vi "transmit.vi"(8 "error in (no error)":errorcluster, 11 "DesktopModbus in":refnum<class "DesktopModbus.lvclass">) -> (0 "error out":errorcluster, 3 "DesktopModbus out":refnum<class "DesktopModbus.lvclass">)   [LabVIEW 2015, in "DesktopModbus.lvclass"]
uses:
  DesktopModbus.lvclass
  Common_RT_Modbus/DataTypes/Frame.ctl
  DesktopModbus.lvclass/DesktopModbus.ctl
  Common_RT_Modbus/RTModbus.lvlib
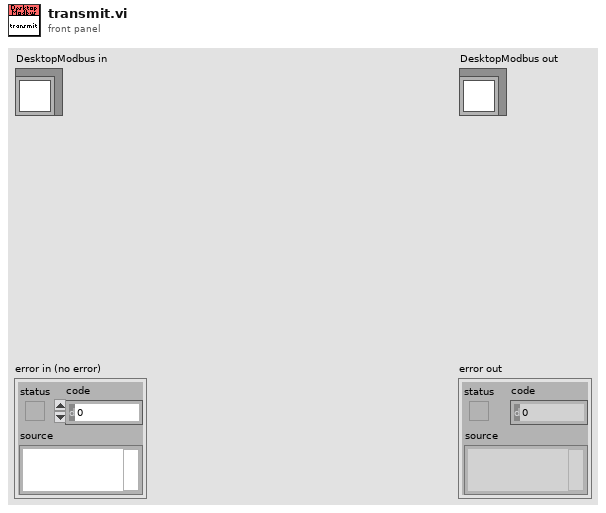
[diagram p1: front panel]
types:
  T1 = typedef "RTModbus.lvlib/Frame.ctl" = cluster{"Data":u8[], "WaitForTrigger":bool, "WaitForRx":u16, "TriggerIRQ":bool, "DelayTicks":u16, "DelayMicroseconds":u16, "DelayMilliseconds":u16}
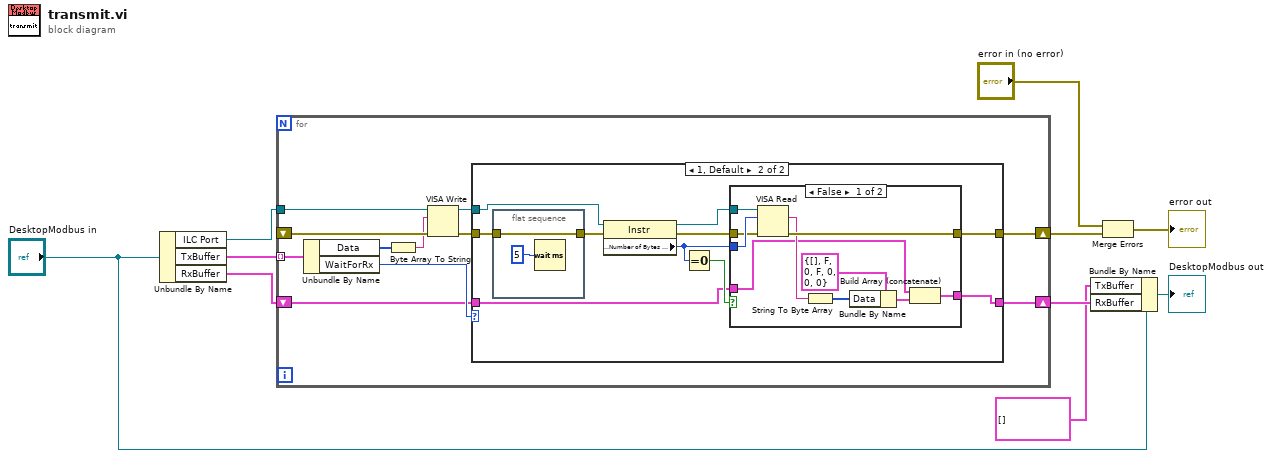
[diagram p0: block diagram]
diagram:
  n1 = Unbundle By Name("DesktopModbus in") -> ("ILC Port"=w9:refnum<visa-resource-name>, "TxBuffer"=w10:T1[], "RxBuffer"=w7:T1[])
  n2 = for {
    tunnel: w10 -> [w19] mode=indexing
    tunnel: w9 -> [w20]
    shift-right: [w14] -> w8
    shift-left: _ -> [w21]
    shift-right: [w11] -> w2
    shift-left: w7 -> [w12]
    n3 = Unbundle By Name(w19) -> ("Data"=w18:u8[], "WaitForRx"=w16:u16)
    n4 = Byte Array To String(unsigned byte array=w18) -> (string=w17:string)
    n5 = VISA Write(VISA resource name=w20, write buffer=w17, error in (no error)=w21) -> (VISA resource name out=w13:refnum<visa-resource-name>, error out=w15:errorcluster)  [unwired: 1 out]
    n6 = case shown="1, Default" w16 {
      tunnel: w15 -> [w23 w33]
      tunnel: [w23 w24] -> w14
      tunnel: w13 -> [_ w32]
      tunnel: w12 -> [w22 w26]
      tunnel: [w22 w25] -> w11
      frame 0 {
      }
      frame 1, Default {
        n7 = flat-sequence {
          tunnel: w33 -> [w46]
          tunnel: [w46] -> w30
          frame #0 {
            n8 = Wait (ms)(milliseconds to wait=u32 5) -> ()  [unwired: 1 out]
          }
        }
        n9 = property class="Instr"(reference=w32, error in=w30) -> (reference out=w31:refnum<visa-resource-name>, error out=w29:errorcluster, "Serial Settings:Number of Bytes at Serial Port"=w27:u32)
        n10 = Equal To 0?(x=w27) -> (x = 0?=w28:bool)
        n11 = case shown="False" w28 {
          tunnel: w27 -> [w43 _]
          tunnel: w31 -> [w42 _]
          tunnel: w29 -> [w41 w45]
          tunnel: [w40 w45] -> w24
          tunnel: w26 -> [w35 w44]
          tunnel: [w34 w44] -> w25
          frame False {
            n12 = VISA Read(VISA resource name=w42, byte count=w43, error in (no error)=w41) -> (read buffer=w37:string, error out=w40:errorcluster)  [unwired: 2 out]
            n13 = String To Byte Array(string=w37) -> (unsigned byte array=w39:u8[])
            n14 = Bundle By Name(cluster=T1 {"Data"=[], "WaitForTrigger"=FALSE, "WaitForRx"=0, "TriggerIRQ"=FALSE, "DelayTicks"=0, "DelayMicroseconds"=0, "DelayMilliseconds"=0} ("Frame"), "Data"=w39) -> (w36:T1)
            n15 = Build Array (concatenate)(w35, w36) -> (w34:T1[])
          }
          frame True {
          }
        }
      }
    }
  }
  n16 = Bundle By Name(cluster="DesktopModbus in", "TxBuffer"=T1[] [], "RxBuffer"=w2) -> (→"DesktopModbus out":refnum<class "DesktopModbus.lvclass">)
  n17 = Merge Errors("error in (no error)", w8) -> (→"error out":errorcluster)
